vi "Read signal out.vi"(8 "error in (no error)":errorcluster, 11 "SignalIn in":refnum<class "SignalIn.lvclass">) -> (0 "error out":errorcluster, 2 "signal out":waveform(dbl)(graph)={"t0"=timestamp(3020748.0 s since 1904-01-01), "dt"=0.001, "Y"=array[1000 elements]}, 3 "SignalIn out":refnum<class "SignalIn.lvclass">)   [LabVIEW 2011, in "SignalIn.lvclass"]
uses:
  SignalIn.lvclass
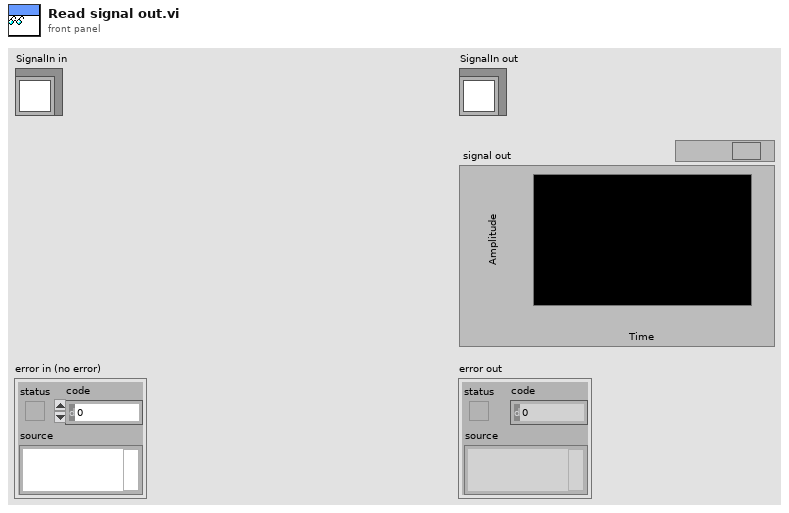
[diagram p1: front panel]
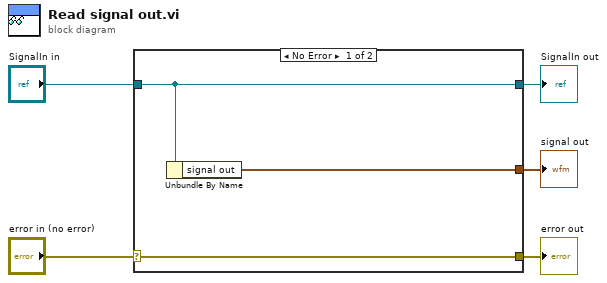
[diagram p0: block diagram]
diagram:
  n1 = case shown="No Error" "error in (no error)" {
    selector: "error in (no error)" -> [w8 w9]
    tunnel: [w8 w9] -> w4
    tunnel: [w7 w10] -> w2
    tunnel: "SignalIn in" -> [w7 w10]
    tunnel: [w6 _] -> w1
    frame No Error {
      n2 = Unbundle By Name(w7) -> ("signal out"=w6:waveform(dbl))
    }
    frame Error {
    }
  }
  "error out" <- w4
  "SignalIn out" <- w2
  "signal out" <- w1
